vi "CompressCircle_Loop.vi"() -> ()   [LabVIEW 2017]
uses:
  Drawing/CircleControls.ctl
  ImageAcquisitionProgram/ImageAcquisitionLibrary/GlobalFrontPanelReferences.vi
  AODControl/AODGlobals.vi
  AODControl/MessageQueue/QueueOperations/Enqueue Message (Single).vi
  ImageAcquisitionProgram/ImageAcquisitionLibrary/ImageAcquisitionLibrary.lvlib
  AODControl/MessageQueue/MessageQueue.lvlib
  AODControl/AODControl.lvlib
panel:
  out "Current Loop":i32
  out "Current Radius":dbl
  in  "N Loops":i32
  in  "input ellipse params":T1={"Radius"=0.0, "No. of Points"=0, "Center"={"X"=0.0, "Y"=0.0}, "Circle"=FALSE, "Density"=0.0, "PointSpec"=enum."No. Of Points", "Hold"=FALSE, "Size"=1, "LatC"=10.0, "Eccentricity"=0.0, "Phase"=0.0} {"Eccentricity" min=0.0; "Size" step=1; "LatC" step=0.05}
  in  "Time (s)":dbl
  in  "Delta R":dbl
  in  "R compressed":dbl
  in  "Exponent":dbl=1.0 format="%#_13g"
  in  "Steps":u32
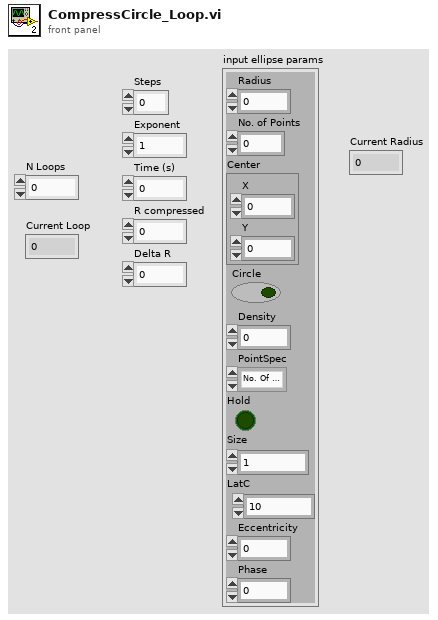
[diagram p1: front panel]
types:
  T1 = typedef "CircleControls.ctl" = cluster{"Radius":dbl, "No. of Points":i32, "Center":cluster{"X":dbl, "Y":dbl}, "Circle":bool, "Density":dbl, "PointSpec":enum32{"No. Of Points", "Density"}, "Hold":bool, "Size":i32, "LatC":dbl, "Eccentricity":dbl, "Phase":dbl}
  T2 = typedef "ImageAcquisitionLibrary.lvlib/References.ctl" = cluster{"Acquire":refnum<vi>, "Rec":refnum<vi>, "Tracking":refnum<vi>, "Settings":refnum<vi>, "Stop":refnum<vi>, "Initialized?":bool, "ImDisplay":refnum<vi>}
  T3 = typedef "AODControl.lvlib/MessageQueue.lvlib/All Message Queues.ctl" = cluster{" AOD Interface":refnum<queue>}
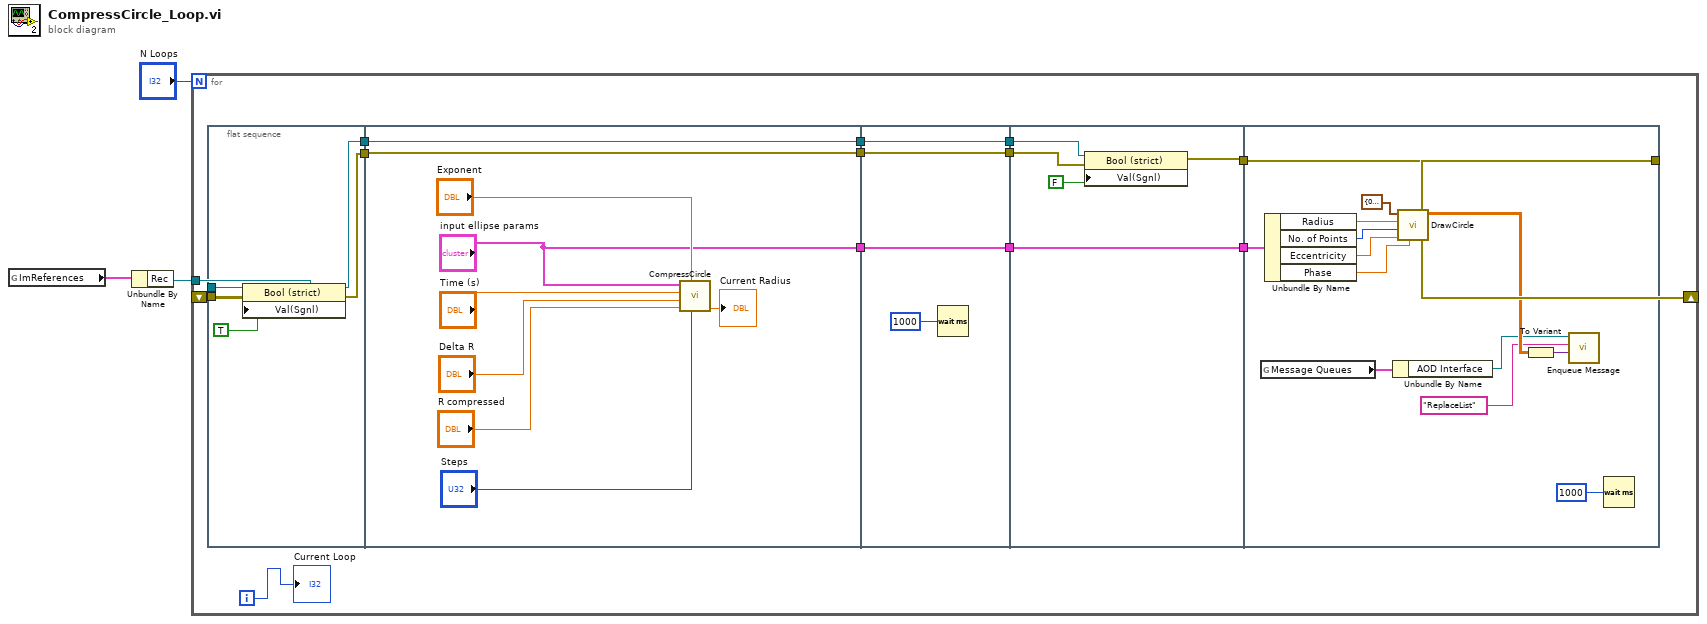
[diagram p0: block diagram]
diagram:
  n1 = global read "GlobalFrontPanelReferences.vi" "ImReferences"() -> (w1:T2)
  n2 = Unbundle By Name(w1) -> ("Rec"=w2:refnum<vi>)
  n3 = for {
    N: "N Loops" -> [_]
    tunnel: w2 -> [w17]
    shift-right: [w12] -> _
    shift-left: _ -> [w16]
    i -> [w10]
    n4 = flat-sequence {
      tunnel: w17 -> [w21]
      tunnel: w16 -> [w20]
      tunnel: [w19] -> w15
      tunnel: [w18] -> w14
      tunnel: [w26] -> w9
      tunnel: w15 -> [w26]
      tunnel: w14 -> [w25]
      tunnel: [w25] -> w7
      tunnel: ["input ellipse params"] -> w5
      tunnel: w9 -> [w35]
      tunnel: [w35] -> w8
      tunnel: w7 -> [w34]
      tunnel: [w34] -> w6
      tunnel: w5 -> [w33]
      tunnel: [w33] -> w4
      tunnel: w8 -> [w40]
      tunnel: w6 -> [w38]
      tunnel: [w37] -> w13
      tunnel: [w36] -> w11
      tunnel: w4 -> [w36]
      tunnel: w13 -> [w52]
      tunnel: [w52] -> w12
      tunnel: w11 -> [w41]
      frame #0 {
        n5 = property class="Bool (strict)"(reference=w21, error in=w20, "Val(Sgnl)"=TRUE ("Value (Signaling)")) -> (reference out=w18:refnum<vi>, error out=w19:errorcluster)
      }
      frame #1 {
        n6 = call "CompressCircle.vi"("Steps"="Steps", "Exponent"="Exponent", "R0"="R compressed", "Delta R"="Delta R", "Time"="Time (s)", "input ellipse params"="input ellipse params") -> ("Current Radius"=→"Current Radius":dbl)  [unwired: 4 in, 1 out]
      }
      frame #2 {
        n7 = Wait (ms)(milliseconds to wait=u32 1000 ("millisecond multiple")) -> ()  [unwired: 1 out]
      }
      frame #3 {
        n8 = property class="Bool (strict)"(reference=w38, error in=w40, "Val(Sgnl)"=FALSE ("Value (Signaling)")) -> (error out=w37:errorcluster)  [unwired: 1 out]
      }
      frame #4 {
        n9 = global read "AODGlobals.vi" "Message Queues"() -> (w43:T3)
        n10 = Unbundle By Name(w41) -> ("Radius"=w44:dbl, "No. of Points"=w50:i32, "Eccentricity"=w46:dbl, "Phase"=w45:dbl)
        n11 = Unbundle By Name(w43) -> ("AOD Interface"=w42:refnum<queue>)
        n12 = call "DrawCircle.vi"("Phase"=w45, "Eccentricity"=w46, "No Of Points"=w50, "Radius"=w44, "Center"=cluster{"X":dbl, "Y":dbl} {"X"=0.0, "Y"=0.0}) -> ("Array"=w49:dbl[][])  [unwired: 6 in]
        n13 = To Variant(anything=w49) -> (Variant=w51:variant)
        n14 = call-poly "Enqueue Message.vi"("Message Data"=w51, "Message"="ReplaceList", "Message Queue"=w42) -> ()  [unwired: 7 in, 2 out]
        n15 = Wait (ms)(milliseconds to wait=u32 1000 ("millisecond multiple")) -> ()  [unwired: 1 out]
      }
    }
    "Current Loop" <- w10
  }
